vi "HardwareOutput.vi"(8 "error in":errorcluster, 9 "Update Outputs":bool, 10 "Motor Control Cluster":T1, 11 "DAQREFs in":T3) -> (0 "error out":errorcluster, 3 "DAQREFs out":T3)   [LabVIEW 2021]
uses:
  Muscle Actuator LabV Analog/Controls/DAQ Refnums.ctl
  TypeDef/MotorControlCluster.ctl
  Muscle Actuator LabV Analog/Controls/Status Lights.ctl
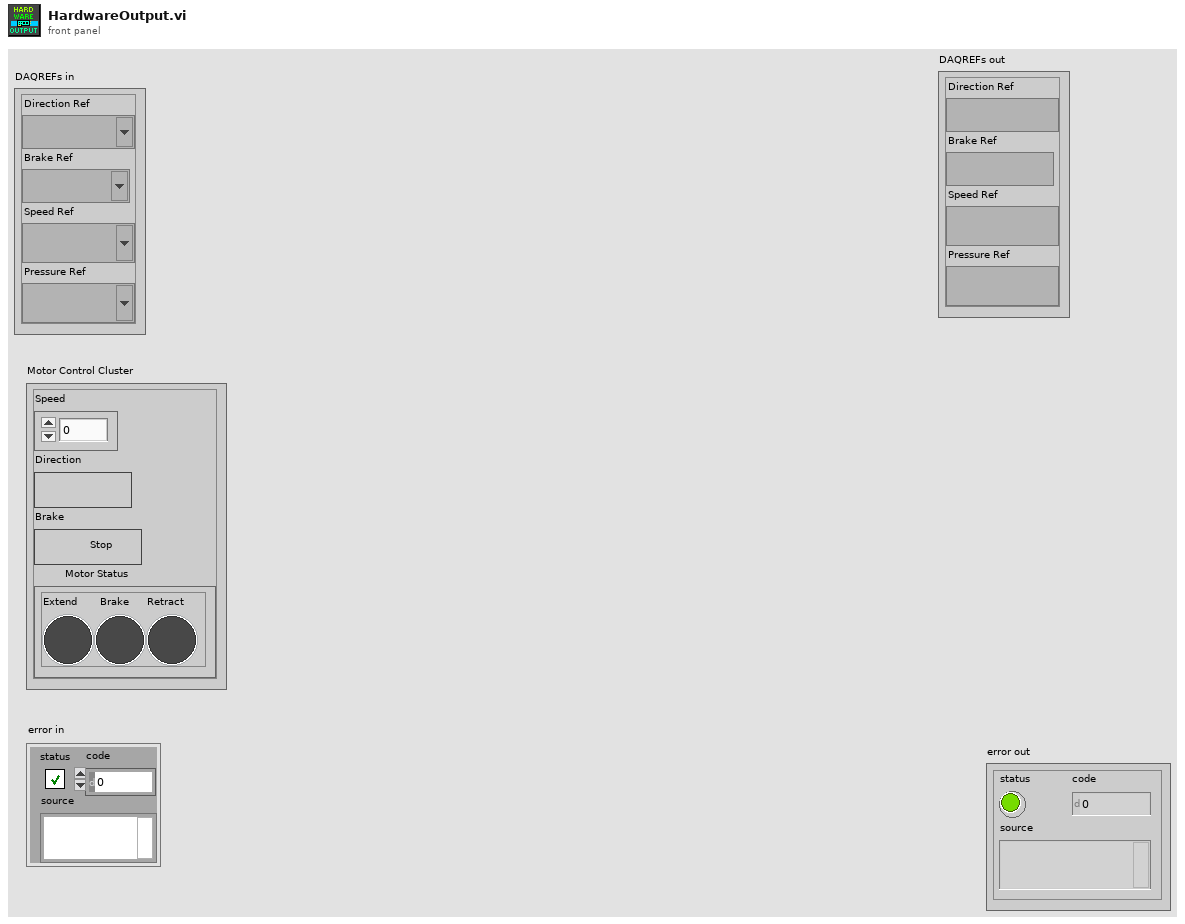
[diagram p1: front panel]
types:
  T1 = typedef "MotorControlCluster.ctl" = cluster{"Speed":dbl, "Direction":bool, "Brake":bool, "Motor Status":T2}
  T2 = typedef "Status Lights.ctl" = cluster{"Extend":bool, "Brake":bool, "Retract":bool}
  T3 = typedef "DAQ Refnums.ctl" = cluster{"Direction Ref":refnum<k21>, "Brake Ref":refnum<k21>, "Speed Ref":refnum<k21>, "Pressure Ref":refnum<k21>}
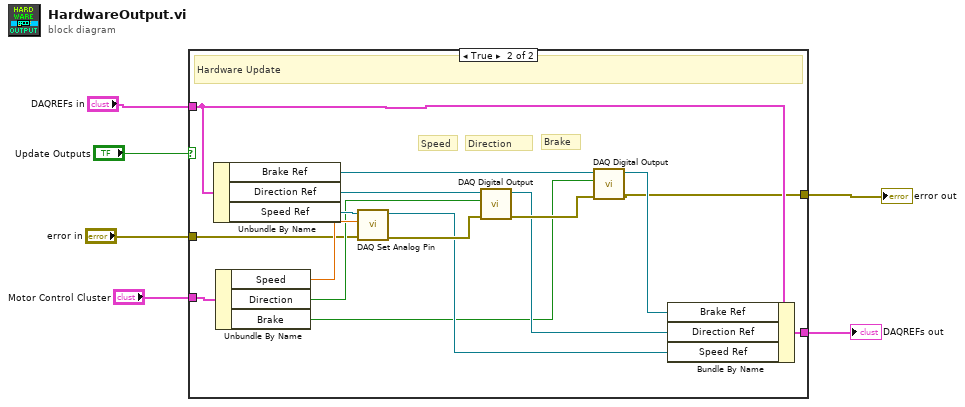
[diagram p0: block diagram]
diagram:
  n1 = case shown="True" "Update Outputs" {
    tunnel: "DAQREFs in" -> [w7 w21]
    tunnel: [w7 w22] -> w6
    tunnel: "Motor Control Cluster" -> [_ w14]
    tunnel: [w8 w10] -> w2
    tunnel: "error in" -> [w8 w9]
    frame False {
      # "No Hardware Update"
    }
    frame True {
      # "Brake"
      # "Direction"
      # "Speed"
      # "Hardware Update"
      n2 = Unbundle By Name(w21) -> ("Brake Ref"=w18:refnum<k21>, "Direction Ref"=w19:refnum<k21>, "Speed Ref"=w20:refnum<k21>)
      n3 = Unbundle By Name(w14) -> ("Speed"=w13:dbl, "Direction"=w12:bool, "Brake"=w11:bool)
      n4 = call "DAQ Set Analog Pin.vi"("error in"=w9, "Voltage"=w13, "task/channels in"=w20) -> ("error out"=w24:errorcluster, "task out"=w17:refnum<k21>)  [unwired: 6 in, 1 out]
      n5 = call "DAQ Digital Output.vi"("error in"=w24, "data"=w12, "task/channels in"=w19) -> ("error out"=w23:errorcluster, "task out"=w16:refnum<k21>)  [unwired: 6 in, 1 out]
      n6 = call "DAQ Digital Output.vi"("error in"=w23, "data"=w11, "task/channels in"=w18) -> ("error out"=w10:errorcluster, "task out"=w15:refnum<k21>)  [unwired: 6 in, 1 out]
      n7 = Bundle By Name(cluster=w21, "Brake Ref"=w15, "Direction Ref"=w16, "Speed Ref"=w17) -> (w22:T3)
    }
  }
  "DAQREFs out" <- w6
  "error out" <- w2
